vi "Quantiser RT Circ.vi"(9 "Objects":T3[](array[typedef]) {"Aspect Ratio" format="%.2f"; "Orientation" format="%.2f"; "Area" format="%.2f"; "Object Center"."Y" format="%.2f"; "Object Center"."X" format="%.2f"}, 10 "INSTR":u8) -> (0 "CKey Out":T1=enum."SOL2", 1 "DKey Out":T2=enum."SOL2", 2 "M 1/L":fxp<+,32,32>, 3 "Punch 1/L":bool, 4 "Gate 1/L":bool, 5 "Gate R":bool, 6 "Trig 1/L":bool, 7 "Trig R":bool)   [LabVIEW 2015]
uses:
  TypeDefs Host/Object Info.ctl
  TypeDefs Host/D major.ctl
  TypeDefs Host/C major.ctl
  TypeDefs Host/Scales.ctl
panel:
  out "Stay R":fxp<+,32,32>
  out "M R":fxp<+,32,32>
  out "Stay 1/L":fxp<+,32,32>
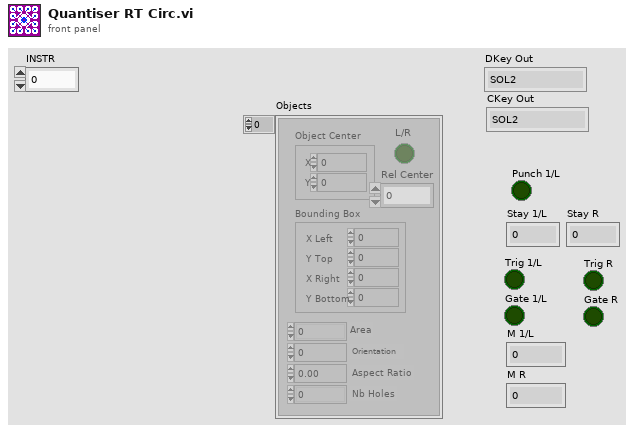
[diagram p1: front panel]
types:
  T1 = typedef "C major.ctl" = enum16{"DO2", "RE2", "MI2", "FA2", "SOL2", "LA2", "SI2", "DO3", "RE3", "MI3", "FA3", "SOL3", "LA3", "SI3"}
  T2 = typedef "D major.ctl" = enum16{"RE2", "MI2", "FA#2", "SOL2", "LA2", "SI2", "DO#3", "RE3", "MI3", "FA#3", "SOL3", "LA3"}
  T3 = typedef "Object Info.ctl" = cluster{"Object Center":cluster{"X":u16, "Y":u16}, "Bounding Box":cluster{"X Left":u16, "Y Top":u16, "X Right":u16, "Y Bottom":u16}, "Area":u16, "Orientation":u16, "Aspect Ratio":sgl, "Nb Holes":u16, "L/R":bool, "Rel Center":u16}
  T4 = typedef "Scales.ctl" = enum16{"ALL", "DO", "RE"}
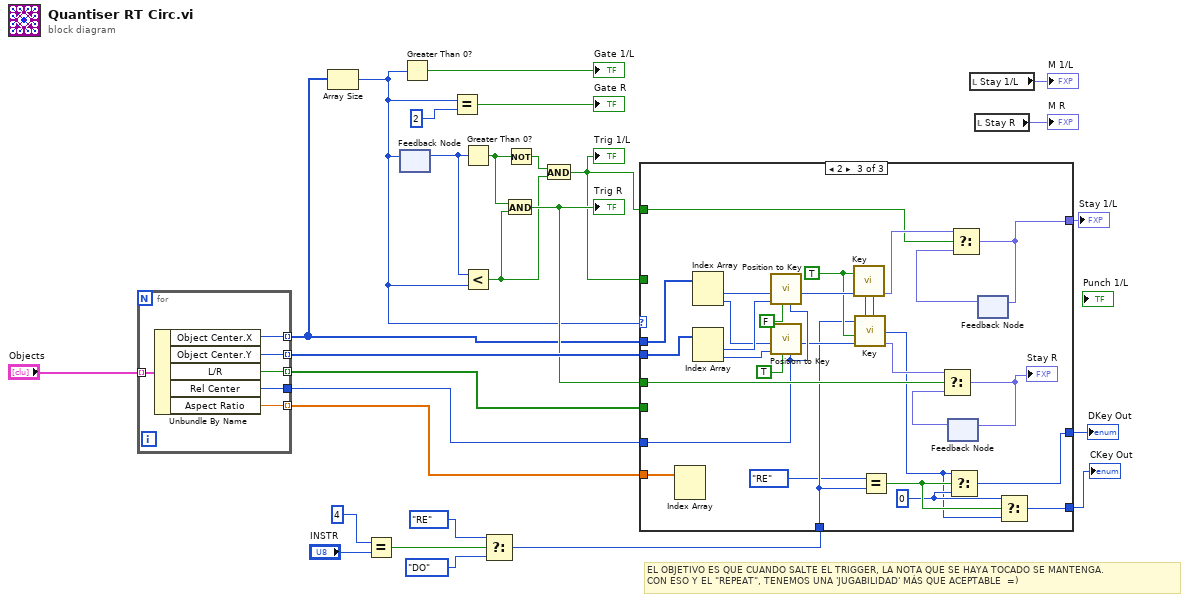
[diagram p0: block diagram]
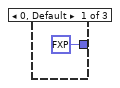
[diagram p2: hidden frame]
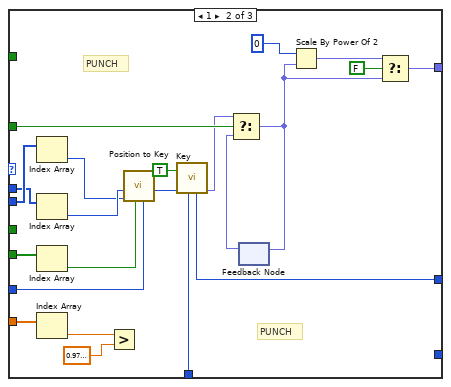
[diagram p3: hidden frame]
diagram:
  # "EL OBJETIVO ES QUE CUANDO SALTE EL TRIGGER, LA NOTA QUE SE HAYA TOCADO SE MANTENGA.\nCON ESO Y EL \"REPEAT\", TENEMOS UNA 'JUGABILIDAD' MÁS QUE ACEPTABLE  =)"
  n1 = for {
    tunnel: "Objects" -> [w33] mode=indexing
    tunnel: [w32] -> w13 mode=indexing
    tunnel: [w31] -> w26 mode=indexing
    tunnel: [w30] -> w12
    tunnel: [w29] -> w11 mode=indexing
    tunnel: [w28] -> w9 mode=indexing
    n2 = Unbundle By Name(w33) -> ("Object Center.X"=w32:u16, "Object Center.Y"=w31:u16, "L/R"=w29:bool, "Rel Center"=w30:u16, "Aspect Ratio"=w28:sgl)
  }
  n3 = Array Size(array=w13) -> (size(s)=w14:i32)
  n4 = Equal?(x=u8 4, y="INSTR") -> (x = y?=w6:bool)
  n5 = feedback #1() -> (w24:i32)  [unwired: 1 in]
  n6 = feedback-in #1(w14) -> ()
  n7 = Greater Than 0?(x=w14) -> (x > 0?=→"Gate 1/L":bool)
  n8 = Equal?(x=w14, y=2) -> (x = y?=→"Gate R":bool)
  n9 = Greater Than 0?(x=w24) -> (x > 0?=w22:bool)
  n10 = Less?(x=w24, y=w14) -> (x < y?=w18:bool)
  n11 = Select(t=Scales."RE" ("Scale"), s=w6, f=Scales."DO" ("Scale")) -> (s? t:f=w3:T4)
  n12 = And(x=w22, y=w18) -> (x .and. y?=w19:bool)
  "Trig R" <- w19
  n13 = Not(x=w22) -> (.not. x?=w20:bool)
  n14 = And(x=w20, y=w18) -> (x .and. y?=w17:bool)
  "Trig 1/L" <- w17
  n15 = case shown="2" w14 {
    tunnel: w13 -> [_ w55 w84]
    tunnel: w26 -> [_ w56 w83]
    tunnel: w17 -> [_ w52 _]
    tunnel: w19 -> [_ _ w74]
    tunnel: w17 -> [_ _ w77]
    tunnel: [fxp<+,32,32> 0.0 ("M") w45 w75] -> w21
    tunnel: w12 -> [_ w49 w70]
    tunnel: w11 -> [_ w47 _]
    tunnel: w9 -> [_ w44 w65]
    tunnel: [_ w37 w61] -> w8
    tunnel: w3 -> [_ w35 w63]
    tunnel: [_ _ w58] -> w1
    frame 0, Default {
    }
    frame 1 {
      # "PUNCH"
      # "PUNCH"
      n16 = Index Array(array=w56) -> (element=w53:u16)  [unwired: 1 in]
      n17 = Index Array(array=w55) -> (element=w54:u16)  [unwired: 1 in]
      n18 = Index Array(array=w47) -> (element=w46:bool)  [unwired: 1 in]
      n19 = Index Array(array=w44) -> (element=w43:sgl)  [unwired: 1 in]
      n20 = Greater?(x=w43, y=sgl 0.97) -> ()  [unwired: 1 out]
      n21 = call "Position to Key.vi"("Rel Center"=w49, "L/R"=w46, "Pos y"=w53, "Pos x"=w54) -> ("Key"=w48:u8)  [unwired: 7 in]
      n22 = call "Key.vi"("Scale"=w35, "Key"=w48, "Enable"=TRUE) -> ("M"=w50:fxp<+,32,32>, "Key out"=w37:u8)  [unwired: 7 in]
      n23 = feedback #2() -> (w51:fxp<+,32,32>)  [unwired: 1 in]
      n24 = Select(t=w50, s=w52, f=w51) -> (s? t:f=w39:fxp<+,32,32>)
      n25 = feedback-in #2(w39) -> ()
      n26 = Scale By Power Of 2(n=i16 0, x=w39) -> (x*2^n=w40:fxp<+,32,32>)
      n27 = Select(t=w40, s=FALSE, f=w39) -> (s? t:f=w45:fxp<+,32,32>)
    }
    frame 2 {
      w59 = u8 0 ("f")
      w64 = TRUE ("Enable")
      n28 = Index Array(array=w65) -> ()  [unwired: 2 in, 2 out]
      n29 = Index Array(array=w84) -> (element #1=w82:u16, element #2=w80:u16)  [unwired: 2 in]
      n30 = Index Array(array=w83) -> (element #1=w81:u16, element #2=w79:u16)  [unwired: 2 in]
      n31 = call "Position to Key.vi"("Rel Center"=w70, "L/R"=FALSE, "Pos y"=w81, "Pos x"=w82) -> ("Key"=w69:u8)  [unwired: 7 in]
      n32 = call "Position to Key.vi"("Rel Center"=w70, "L/R"=TRUE, "Pos y"=w79, "Pos x"=w80) -> ("Key"=w68:u8)  [unwired: 7 in]
      n33 = call "Key.vi"("Scale"=w63, "Key"=w69, "Enable"=w64) -> ("M"=w78:fxp<+,32,32>, "Key out"=w57:u8)  [unwired: 7 in]
      n34 = call "Key.vi"("Scale"=w63, "Key"=w68, "Enable"=w64) -> ("M"=w73:fxp<+,32,32>)  [unwired: 7 in, 1 out]
      n35 = Equal?(x=Scales."RE" ("Scale"), y=w63) -> (x = y?=w60:bool)
      n36 = feedback #3() -> (w71:fxp<+,32,32>)  [unwired: 1 in]
      n37 = Select(t=w73, s=w74, f=w71) -> (s? t:f=w72:fxp<+,32,32>)
      "Stay R" <- w72
      n38 = feedback-in #3(w72) -> ()
      n39 = Select(t=w57, s=w60, f=w59) -> (s? t:f=w61:u8)
      n40 = feedback #4() -> (w76:fxp<+,32,32>)  [unwired: 1 in]
      n41 = Select(t=w78, s=w77, f=w76) -> (s? t:f=w75:fxp<+,32,32>)
      n42 = feedback-in #4(w75) -> ()
      n43 = Select(t=w59, s=w60, f=w57) -> (s? t:f=w58:u8)
    }
  }
  "Stay 1/L" <- w21
  "DKey Out" <- w8
  "CKey Out" <- w1
  n44 = local read "Stay 1/L"() -> (→"M 1/L":fxp<+,32,32>)
  n45 = local read "Stay R"() -> (→"M R":fxp<+,32,32>)
